vi "DMA.Wait for Done Interrupt Event.vi"(8 "error in (no error)":errorcluster, 10 "timeout ms (1000)":u32=1000, 11 "GE 5565PIORC":refnum<class "GE 5565PIORC.lvclass">) -> (0 "error out":errorcluster, 2 "Timed out?":bool, 3 "GE 5565PIORC out":refnum<class "GE 5565PIORC.lvclass">)   [LabVIEW 2016, in "GE 5565PIORC.lvclass"]
uses:
  GE 5565PIORC.lvclass
  GE 5565PIORC.lvclass/GE 5565PIORC.ctl
  <vilib>/Utility/error.llb/Clear Errors.vi
  Binary Operations/Set Bits.vi
  Binary Operations/Set Bits U32.vi
  Registers/Local Configuration.Get Register Offset.vi
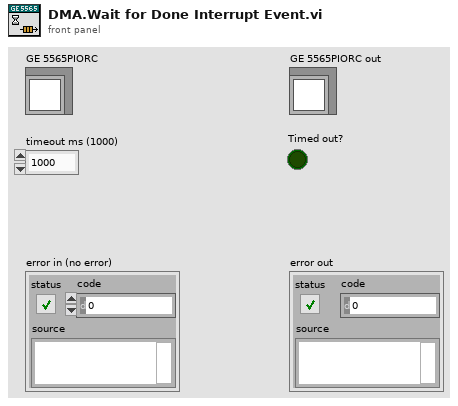
[diagram p1: front panel]
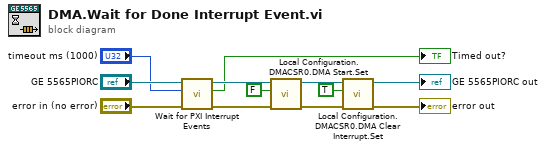
[diagram p0: block diagram]
diagram:
  n1 = call "Wait for PXI Interrupt Events.vi"("error in (no error)"="error in (no error)", "timeout ms (1000)"="timeout ms (1000)", "GE 5565PIORC in"="GE 5565PIORC") -> ("error out"=w9:errorcluster, "Timed out?"=→"Timed out?":bool, "GE 5565PIORC out"=w5:refnum<class "GE 5565PIORC.lvclass">)  [unwired: 6 in]
  n2 = call "Local Configuration.DMACSR0.DMA Start.Set.vi"("error in (no error)"=w9, "Start DMA?"=FALSE, "GE 5565PIORC"=w5) -> ("error out"=w8:errorcluster, "GE 5565PIORC out"=w6:refnum<class "GE 5565PIORC.lvclass">)  [unwired: 7 in]
  n3 = call "Local Configuration.DMACSR0.DMA Clear Interrupt.Set.vi"("error in (no error)"=w8, "Clear Interrupt?"=TRUE, "GE 5565PIORC"=w6) -> ("error out"=→"error out":errorcluster, "GE 5565PIORC out"=→"GE 5565PIORC out":refnum<class "GE 5565PIORC.lvclass">)  [unwired: 7 in]
